vi "searchModulePath.vi"(8 "error in (no error)":errorcluster) -> (0 "error out":errorcluster, 2 "module path out":path)   [LabVIEW 2022 SP3, in "openDAQ.lvlib"]
uses:
  openDAQ.lvlib
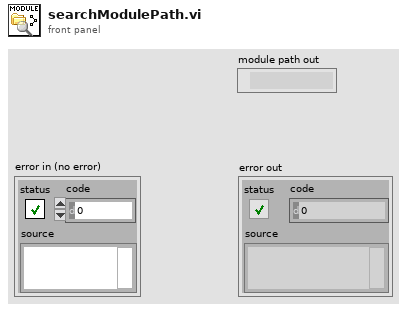
[diagram p1: front panel]
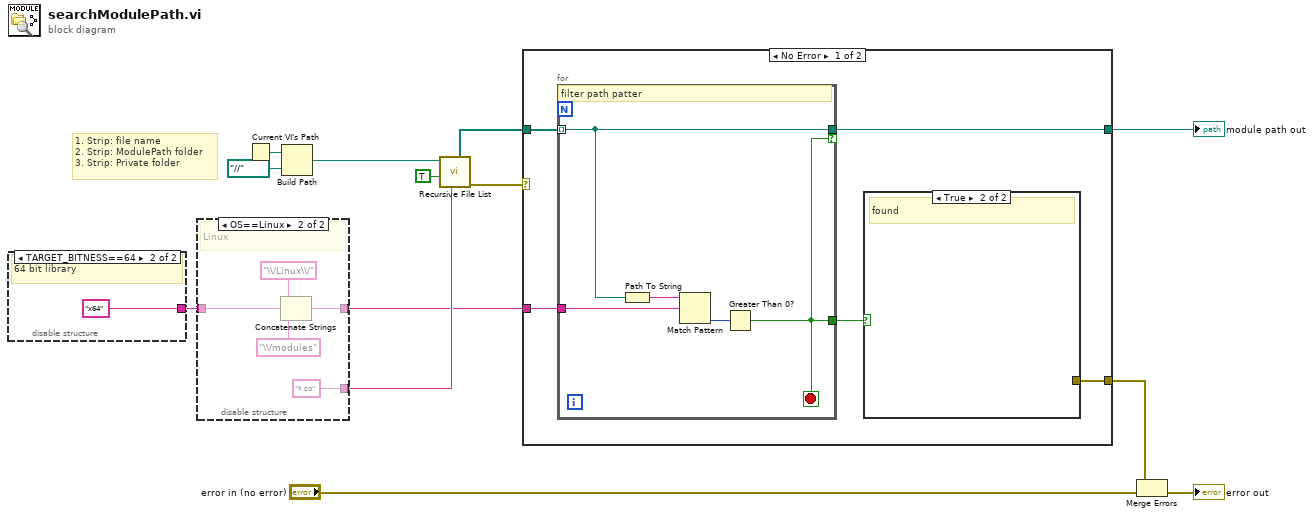
[diagram p0: block diagram]
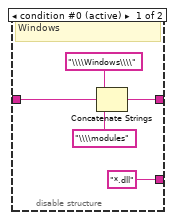
[diagram p2: hidden frame]
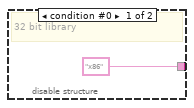
[diagram p3: hidden frame]
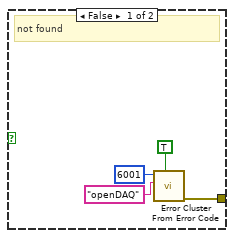
[diagram p4: hidden frame]
diagram:
  # "1. Strip: file name\n2. Strip: ModulePath folder\n3. Strip: Private folder"
  n1 = disable-structure shown="TARGET_BITNESS==64" {
    disable-tunnel: ["x86" "x64"] -> w3
    frame condition #0 {
      # "32 bit library"
    }
    frame condition #1 (active) {
      # "64 bit library"
    }
  }
  n2 = disable-structure shown="OS==Linux" {
    disable-tunnel: w3 -> [w19 w24]
    disable-tunnel: [w17 w22] -> w8
    disable-tunnel: ["*.dll" "*.so"] -> w13
    frame condition #0 (active) {
      # "Windows"
      n3 = Concatenate Strings("\\\\Windows\\\\", w19, "\\\\modules") -> (w17:string)
    }
    frame condition #1 {
      # "Linux"
      n4 = Concatenate Strings("\\/Linux\\/", w24, "\\/modules") -> (w22:string)
    }
  }
  n5 = Current VI's Path() -> (path=w2:path)
  n6 = Build Path(base path=w2, name or relative path=path "../../..") -> (appended path=w12:path)
  n7 = call <vilib>:"Recursive File List.vi"("pattern"=w13, "Continue Recursing on Error? (F)"=TRUE, "Folder Path"=w12) -> ("error out"=w10:errorcluster, "All Folders"=w9:path[])  [unwired: 4 in, 3 out]
  n8 = case shown="No Error" w10 {
    selector: w10 -> [_ w40]
    tunnel: w9 -> [w30 _]
    tunnel: w8 -> [w29 _]
    tunnel: [w28 _] -> w7
    tunnel: [w26 w40] -> w6
    frame No Error {
      n9 = for {
        tunnel: w30 -> [w35] mode=indexing
        tunnel: [w35] -> w28 if=w31
        tunnel: w29 -> [w33]
        tunnel: [w31] -> w27
        stop <- w31 stop-if-true
        # "filter path patter"
        n10 = Path To String(path=w35) -> (string=w34:string)
        n11 = Match Pattern(string=w34, regular expression=w33) -> (offset past match=w32:i32)  [unwired: 1 in, 3 out]
        n12 = Greater Than 0?(x=w32) -> (x > 0?=w31:bool)
      }
      n13 = case shown="True" w27 {
        tunnel: [w36 _] -> w26
        frame False {
          # "not found"
          n14 = call <vilib>:"Error Cluster From Error Code.vi"("show call chain? (False)"=TRUE, "error message (\"\")"="openDAQ" ("error message (\"\")"), "error code (0)"=6001) -> ("error out"=w36:errorcluster)  [unwired: 6 in]
        }
        frame True {
          # "found"
        }
      }
    }
    frame Error {
    }
  }
  "module path out" <- w7
  n15 = Merge Errors(w6, "error in (no error)") -> (→"error out":errorcluster)
